vi "runDisplay.vi"(8 "error in (no error)":errorcluster, 11 "Display":refnum<class "StatisticsDisplay.lvclass">) -> (0 "error out":errorcluster, 3 "Display":refnum<class "StatisticsDisplay.lvclass">)   [LabVIEW 2020, in "StatisticsDisplay.lvclass"]
uses:
  StatisticsDisplay.lvclass
  C:/Projects/Repos/HeadFirstDesignPatterns/HeadFirstDesignPatternsLabVIEWandPython/02 Observer/LabVIEW/DisplayBase/DisplayBase.lvclass
  StatisticsDisplay.lvclass/StatisticsDisplay.ctl
  DisplayBase/DisplayBase.lvclass
panel:
  out "Min":dbl(slide) scale=0.0..100.0
  out "Average":dbl(slide) scale=0.0..100.0
  out "Max":dbl(slide) scale=0.0..100.0
  # "Temperature Statistics"
  # "Connector Pane"
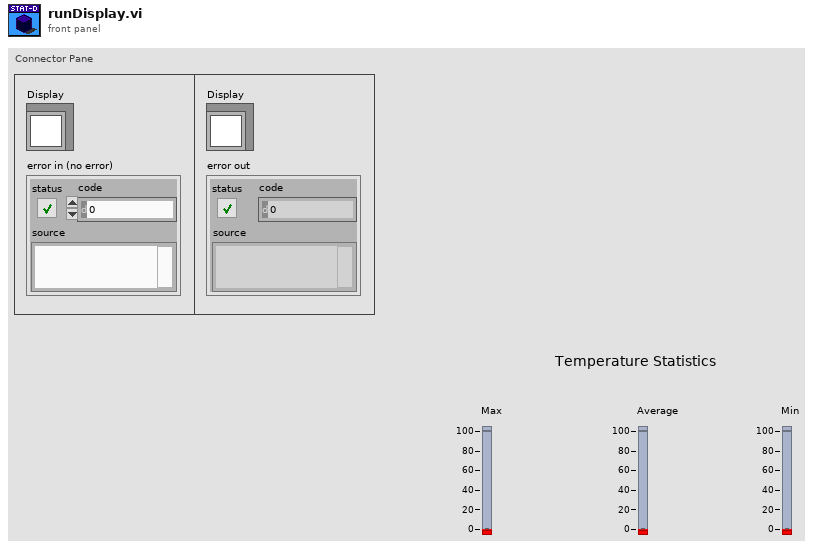
[diagram p1: front panel]
types:
  T1 = typedef "StatisticsDisplay.lvclass/StatisticsData.ctl" = cluster{"maxTemp":dbl, "minTemp":dbl, "TempSum":dbl, "nReadings":i32}
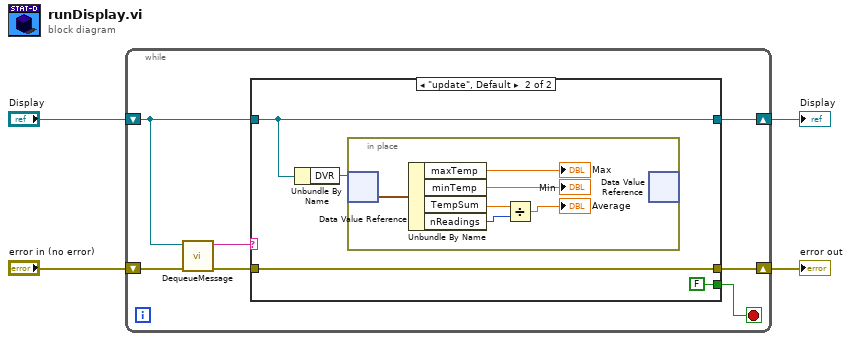
[diagram p0: block diagram]
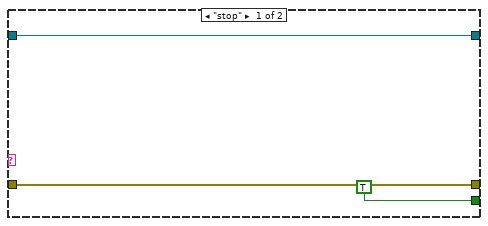
[diagram p2: hidden frame]
diagram:
  n1 = while {
    shift-right: [w11] -> w3
    shift-left: "error in (no error)" -> [w8]
    shift-right: [w10] -> w4
    shift-left: "Display" -> [w7]
    stop <- w9 stop-if-true
    n2 = call "DequeueMessage.vi"("error in (no error)"=w8, "DisplayBase in"=w7) -> ("error out"=w6:errorcluster, "String"=w5:string)  [unwired: 8 in]
    n3 = case shown="\"update\", Default" w5 {
      tunnel: w7 -> [w12 w16]
      tunnel: w6 -> [w14 w18]
      tunnel: [w14 w18] -> w11
      tunnel: [w12 w16] -> w10
      tunnel: [TRUE FALSE] -> w9
      frame "stop" {
      }
      frame "update", Default {
        n4 = Unbundle By Name(w16) -> ("DVR"=w15:refnum<data-value>)
        n5 = in-place {
          n6 = in-place-dvr #1(w15) -> (w24:T1)  [unwired: 1 out]
          n7 = Unbundle By Name(w24) -> ("maxTemp"=→"Max":dbl, "minTemp"=→"Min":dbl, "TempSum"=w21:dbl, "nReadings"=w20:i32)
          n8 = Divide(x=w21, y=w20) -> (x/y=→"Average":dbl)
          n9 = in-place-dvr #1() -> ()  [unwired: 1 in, 2 out]
        }
      }
    }
  }
  "Display" <- w4
  "error out" <- w3
